vi "Select Ball By Confidence.vi"(10 "Array":T1[](array[typedef]) {"robots_blue"."height" format="%+4.3f"; "robots_blue"."pixel_y" format="%+4.3f"; "robots_blue"."pixel_x" format="%+4.3f"; "robots_blue"."orientation" format="%+4.3f"; "robots_blue"."y" format="%+4.3f"; "robots_blue"."confidence" format="%4.3f"; "robots_blue"."x" format="%+4.3f"; "robots_yellow"."height" format="%+4.3f"; "robots_yellow"."pixel_y" format="%+4.3f"; "robots_yellow"."pixel_x" format="%+4.3f"; "robots_yellow"."orientation" format="%+4.3f"; "robots_yellow"."y" format="%+4.3f"; "robots_yellow"."confidence" format="%4.3f"; "robots_yellow"."x" format="%+4.3f"}, 11 "balls":T4[](array[typedef])) -> (3 "balls out":T4[](array[typedef]))   [LabVIEW 2017]
uses:
  <vilib>/Analysis/Matrix/Datatypes/RealMatrix.ctl
  <vilib>/Analysis/Matrix/NI_Matrix.lvlib
  SSL Detection Ball.ctl
  SSL Detection Robot.ctl
  SSL Detection Frame.ctl
panel:
  in  "Boolean":bool
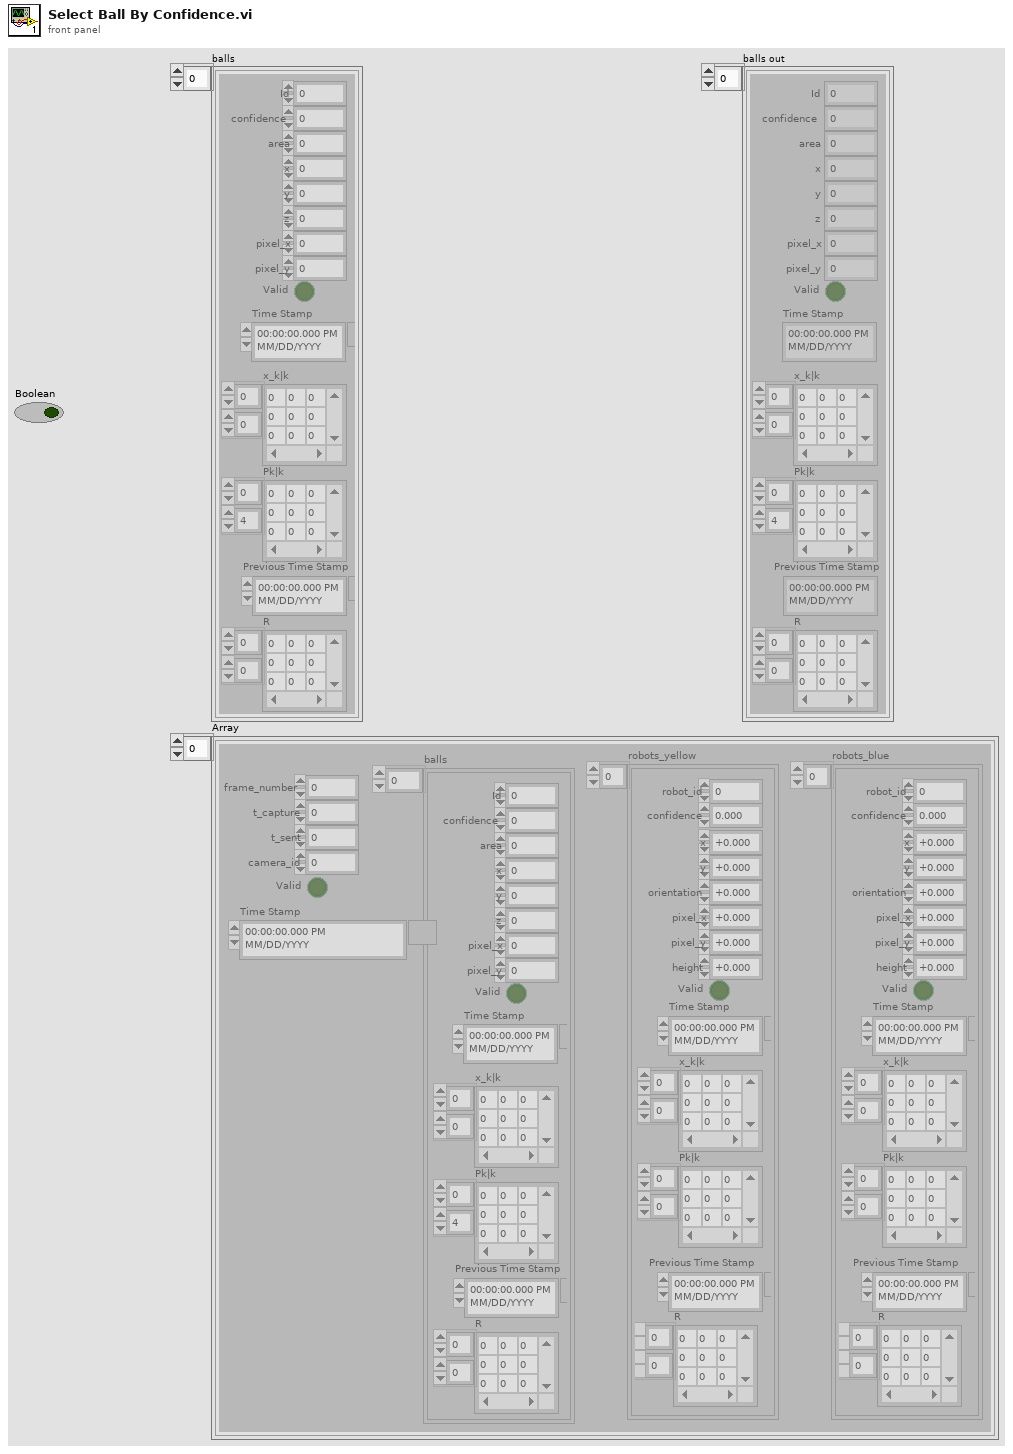
[diagram p1: front panel]
types:
  T1 = typedef "SSL Detection Frame.ctl" = cluster{"frame_number":u32, "t_capture":dbl, "t_sent":dbl, "camera_id":u32, "robots_yellow":T2[], "robots_blue":T2[], "balls":T4[], "Valid":bool, "Time Stamp":timestamp}
  T2 = typedef "SSL Detection Robot.ctl" = cluster{"x":sgl, "robot_id":u32, "confidence":sgl, "y":sgl, "orientation":sgl, "pixel_x":sgl, "pixel_y":sgl, "height":sgl, "Valid":bool, "Time Stamp":timestamp, "x_k|k":T3, "Pk|k":T3, "Previous Time Stamp":timestamp, "R":T3}
  T3 = typedef "NI_Matrix.lvlib/RealMatrix.ctl" = dbl[][]
  T4 = typedef "SSL Detection Ball.ctl" = cluster{"x":sgl, "area":u32, "confidence":sgl, "y":sgl, "z":sgl, "pixel_x":sgl, "pixel_y":sgl, "Valid":bool, "Time Stamp":timestamp, "x_k|k":T3, "Pk|k":T3, "Id":u32, "Previous Time Stamp":timestamp, "R":T3}
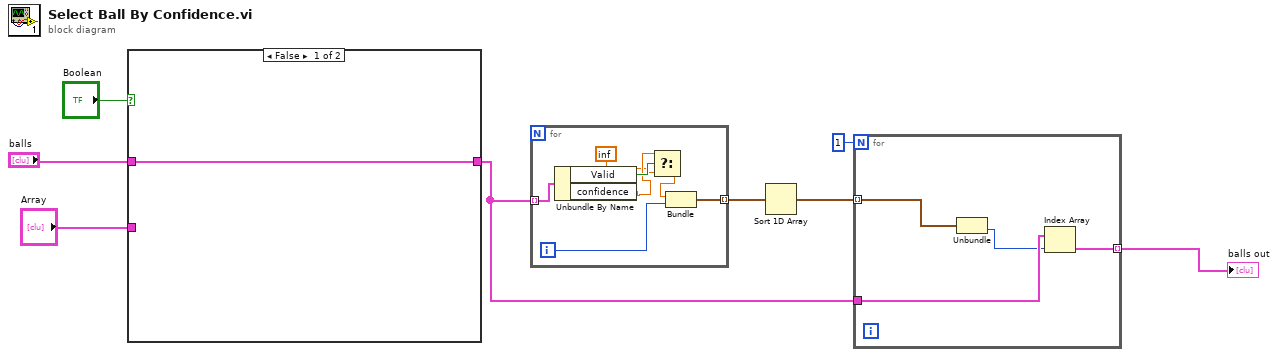
[diagram p0: block diagram]
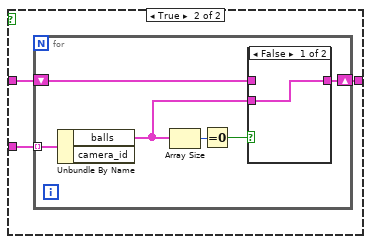
[diagram p2: hidden frame]
diagram:
  n1 = case shown="False" "Boolean" {
    tunnel: "Array" -> [_ w12]
    tunnel: [w9 w11] -> w3
    tunnel: "balls" -> [w9 w10]
    frame False {
    }
    frame True {
      n2 = for {
        tunnel: w12 -> [w18] mode=indexing
        shift-right: [w15] -> w11
        shift-left: w10 -> [w13]
        n3 = Unbundle By Name(w18) -> ("balls"=w14:T4[])  [unwired: 1 out]
        n4 = Array Size(array=w14) -> (size(s)=w17:i32)
        n5 = Equal To 0?(x=w17) -> (x = 0?=w16:bool)
        n6 = case shown="False" w16 {
          tunnel: [w19 w20] -> w15
          tunnel: w14 -> [w19 _]
          tunnel: w13 -> [_ w20]
          frame False {
          }
          frame True {
          }
        }
      }
    }
  }
  n7 = for {
    tunnel: w3 -> [w27] mode=indexing
    tunnel: [w26] -> w8 mode=indexing
    i -> [w25]
    n8 = Unbundle By Name(w27) -> ("Valid"=w24:bool, "confidence"=w23:sgl)
    n9 = Select(t=w23, s=w24, f=inf) -> (s? t:f=w22:dbl)
    n10 = Bundle("confidence"=w22, w25) -> (w26:cluster{"confidence":dbl, i32})  [unwired: 1 in]
  }
  n11 = Sort 1D Array(array=w8) -> (sorted array=w7:cluster{"confidence":dbl, i32}[])
  n12 = for {
    N: 1 -> [_]
    tunnel: w7 -> [w31] mode=indexing
    tunnel: w3 -> [w30]
    tunnel: [w28] -> w6 mode=indexing
    n13 = Unbundle(w31) -> (w29:i32)  [unwired: 1 out]
    n14 = Index Array(array=w30, index=w29) -> (element=w28:T4)
  }
  "balls out" <- w6
